vi "traitement cam A1.vi"(0 "ROI Carré 1":T1={"Global Rectangle"=[636, 369, 672, 405], "Contours"=[{"ID"=enum."External", "Type"=3, "Coordinates"=[636, 369, 672, 405]}]} {"Contours"."Type" items=["No Selection", "Point", "Line", "Rectangle", "Oval", "Polygon", "Freehand Region", "Annulus", "Unused2", "Unused3", "Broken Line", "Freehand Line", "Rotated Rectangle"]}, 7 "error in":errorcluster) -> (20 "Couleur carré 1":string[](array[string]), 27 "error out":errorcluster)   [LabVIEW 2019]
uses:
  <vilib>/vision/Classification.llb/IMAQ Classifier Read Options.ctl
  <vilib>/vision/NI_Vision_Development_Module.lvlib
panel:
  out "Couleur carré 12":string[](array[string])
  out "Couleur carré 11":string[](array[string])
  out "Couleur carré 10":string[](array[string])
  out "Couleur carré 9":string[](array[string])
  out "Couleur carré 8":string[](array[string])
  out "Couleur carré 7":string[](array[string])
  out "Couleur carré 6":string[](array[string])
  out "Couleur carré 5":string[](array[string])
  out "Couleur carré 4":string[](array[string])
  out "Couleur carré 3":string[](array[string])
  out "Couleur carré 2":string[](array[string])
  in  "ROI Carré 12":T1={"Global Rectangle"=[636, 369, 672, 405], "Contours"=[{"ID"=enum."External", "Type"=3, "Coordinates"=[636, 369, 672, 405]}]} {"Contours"."Type" items=["No Selection", "Point", "Line", "Rectangle", "Oval", "Polygon", "Freehand Region", "Annulus", "Unused2", "Unused3", "Broken Line", "Freehand Line", "Rotated Rectangle"]}
  in  "ROI Carré 11":T1={"Global Rectangle"=[636, 369, 672, 405], "Contours"=[{"ID"=enum."External", "Type"=3, "Coordinates"=[636, 369, 672, 405]}]} {"Contours"."Type" items=["No Selection", "Point", "Line", "Rectangle", "Oval", "Polygon", "Freehand Region", "Annulus", "Unused2", "Unused3", "Broken Line", "Freehand Line", "Rotated Rectangle"]}
  in  "ROI Carré 10":T1={"Global Rectangle"=[636, 369, 672, 405], "Contours"=[{"ID"=enum."External", "Type"=3, "Coordinates"=[636, 369, 672, 405]}]} {"Contours"."Type" items=["No Selection", "Point", "Line", "Rectangle", "Oval", "Polygon", "Freehand Region", "Annulus", "Unused2", "Unused3", "Broken Line", "Freehand Line", "Rotated Rectangle"]}
  in  "ROI Carré 9":T1={"Global Rectangle"=[636, 369, 672, 405], "Contours"=[{"ID"=enum."External", "Type"=3, "Coordinates"=[636, 369, 672, 405]}]} {"Contours"."Type" items=["No Selection", "Point", "Line", "Rectangle", "Oval", "Polygon", "Freehand Region", "Annulus", "Unused2", "Unused3", "Broken Line", "Freehand Line", "Rotated Rectangle"]}
  in  "ROI Carré 8":T1={"Global Rectangle"=[636, 369, 672, 405], "Contours"=[{"ID"=enum."External", "Type"=3, "Coordinates"=[636, 369, 672, 405]}]} {"Contours"."Type" items=["No Selection", "Point", "Line", "Rectangle", "Oval", "Polygon", "Freehand Region", "Annulus", "Unused2", "Unused3", "Broken Line", "Freehand Line", "Rotated Rectangle"]}
  in  "ROI Carré 7":T1={"Global Rectangle"=[636, 369, 672, 405], "Contours"=[{"ID"=enum."External", "Type"=3, "Coordinates"=[636, 369, 672, 405]}]} {"Contours"."Type" items=["No Selection", "Point", "Line", "Rectangle", "Oval", "Polygon", "Freehand Region", "Annulus", "Unused2", "Unused3", "Broken Line", "Freehand Line", "Rotated Rectangle"]}
  in  "ROI Carré 6":T1={"Global Rectangle"=[636, 369, 672, 405], "Contours"=[{"ID"=enum."External", "Type"=3, "Coordinates"=[636, 369, 672, 405]}]} {"Contours"."Type" items=["No Selection", "Point", "Line", "Rectangle", "Oval", "Polygon", "Freehand Region", "Annulus", "Unused2", "Unused3", "Broken Line", "Freehand Line", "Rotated Rectangle"]}
  in  "ROI Carré 5":T1={"Global Rectangle"=[636, 369, 672, 405], "Contours"=[{"ID"=enum."External", "Type"=3, "Coordinates"=[636, 369, 672, 405]}]} {"Contours"."Type" items=["No Selection", "Point", "Line", "Rectangle", "Oval", "Polygon", "Freehand Region", "Annulus", "Unused2", "Unused3", "Broken Line", "Freehand Line", "Rotated Rectangle"]}
  in  "ROI Carré 4":T1={"Global Rectangle"=[636, 369, 672, 405], "Contours"=[{"ID"=enum."External", "Type"=3, "Coordinates"=[636, 369, 672, 405]}]} {"Contours"."Type" items=["No Selection", "Point", "Line", "Rectangle", "Oval", "Polygon", "Freehand Region", "Annulus", "Unused2", "Unused3", "Broken Line", "Freehand Line", "Rotated Rectangle"]}
  in  "ROI Carré 3":T1={"Global Rectangle"=[636, 369, 672, 405], "Contours"=[{"ID"=enum."External", "Type"=3, "Coordinates"=[636, 369, 672, 405]}]} {"Contours"."Type" items=["No Selection", "Point", "Line", "Rectangle", "Oval", "Polygon", "Freehand Region", "Annulus", "Unused2", "Unused3", "Broken Line", "Freehand Line", "Rotated Rectangle"]}
  in  "ROI Carré 2":T1={"Global Rectangle"=[636, 369, 672, 405], "Contours"=[{"ID"=enum."External", "Type"=3, "Coordinates"=[636, 369, 672, 405]}]} {"Contours"."Type" items=["No Selection", "Point", "Line", "Rectangle", "Oval", "Polygon", "Freehand Region", "Annulus", "Unused2", "Unused3", "Broken Line", "Freehand Line", "Rotated Rectangle"]}
  out "Image Out":T2(plugin-control)
  # "C\nE\nN\nT\nR\nE\n\nR\nO\nU\nG\nE\nE"
  # "C\nE\nN\nT\nR\nE\n\nB\nL\nA\nN\nC"
  # "C\nE\nN\nT\nR\nE\n\nB\nL\nE\nU"
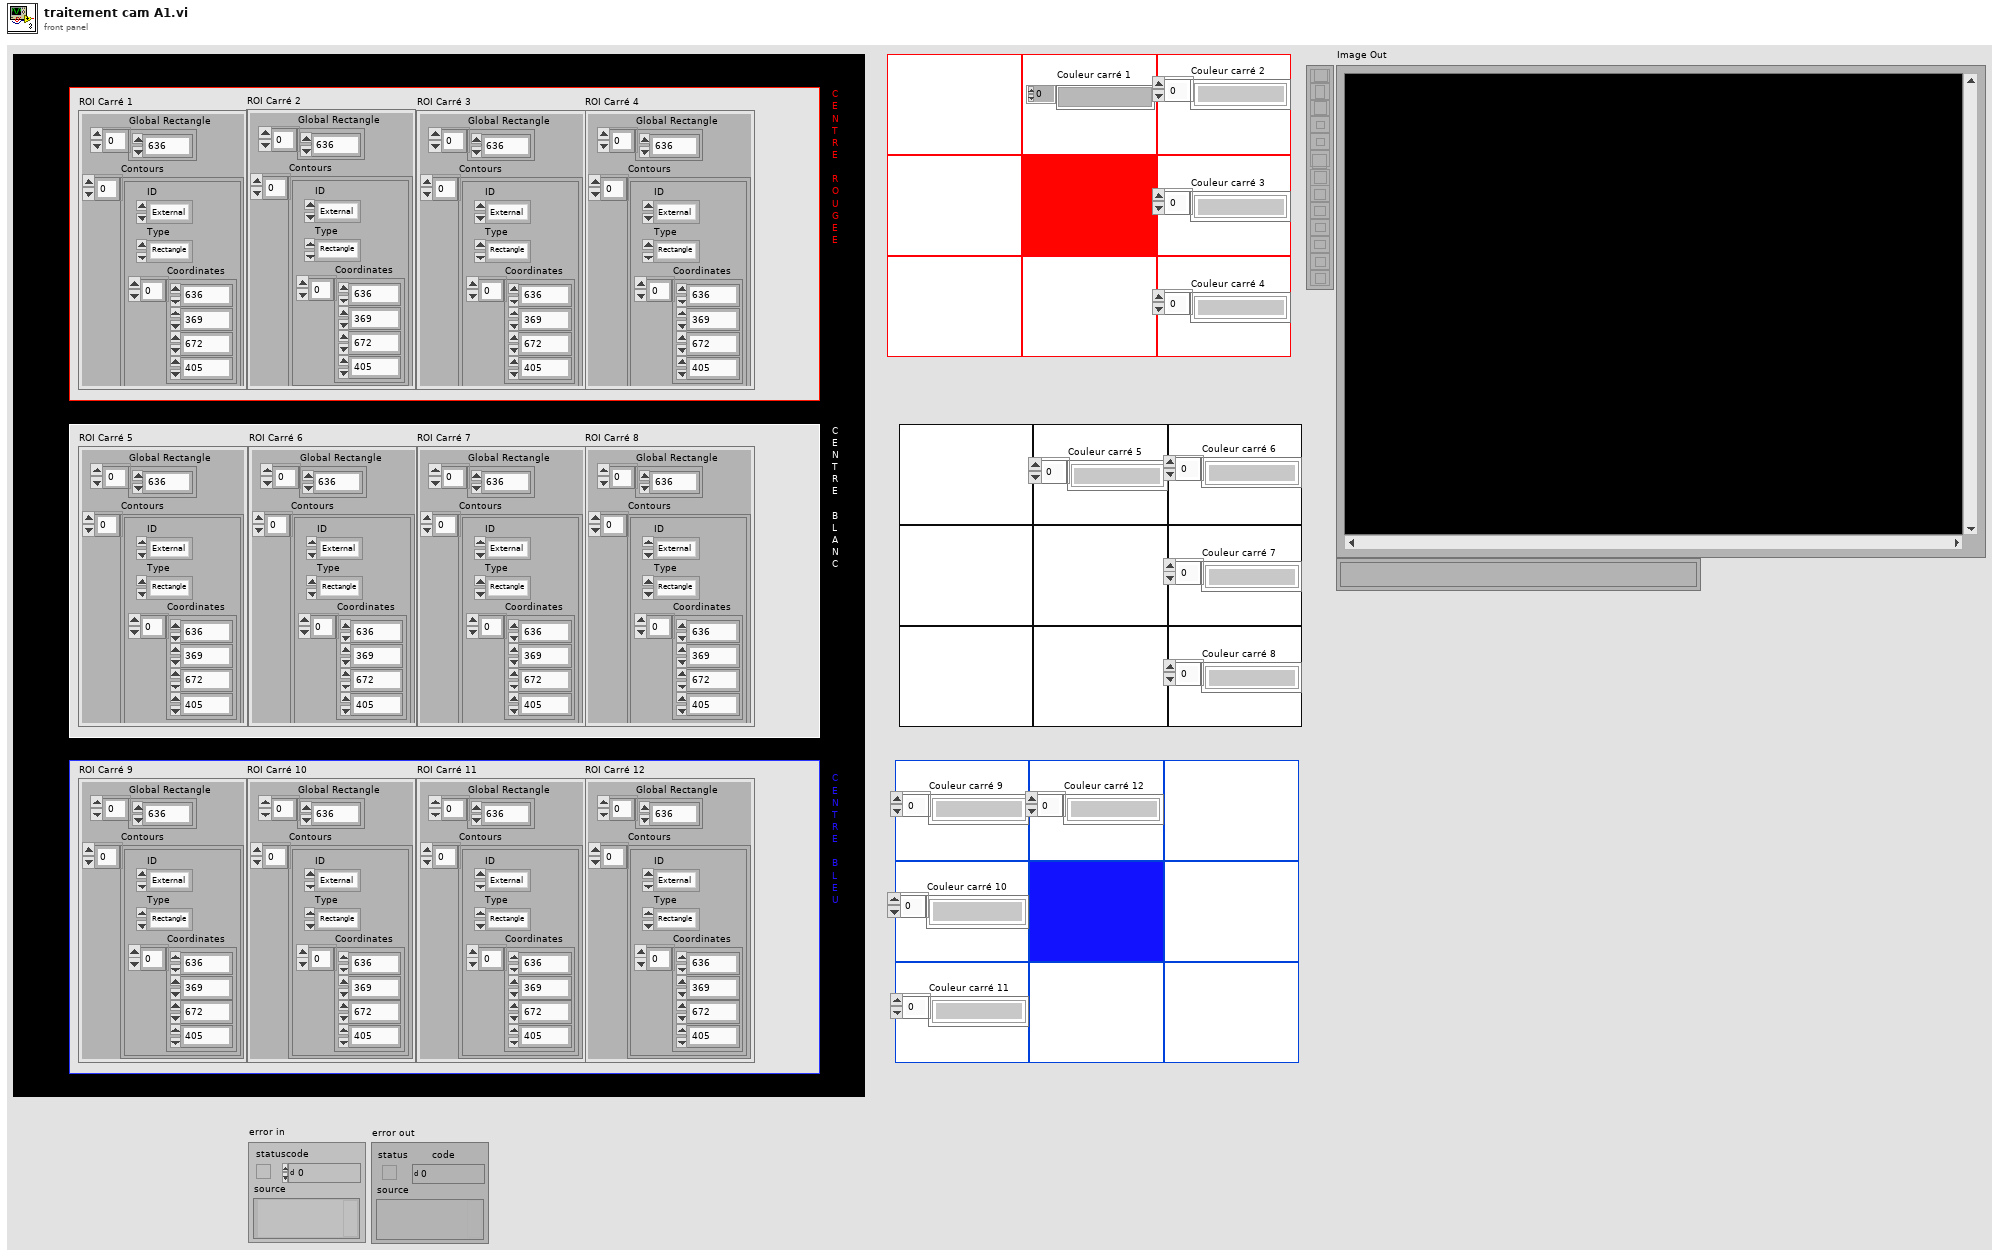
[diagram p1: front panel]
types:
  T1 = cluster{"Global Rectangle":i32[], "Contours":cluster{"ID":enum32{"External", "Internal"}, "Type":u32, "Coordinates":i32[]}[]}
  T2 = typedef "IMAQ Image.ctl" = refnum<image>
  T3 = typedef "IMAQ Classifier Read Options.ctl" = i32
  T4 = typedef "IMAQ Classifier Session.ctl" = refnum<k1>
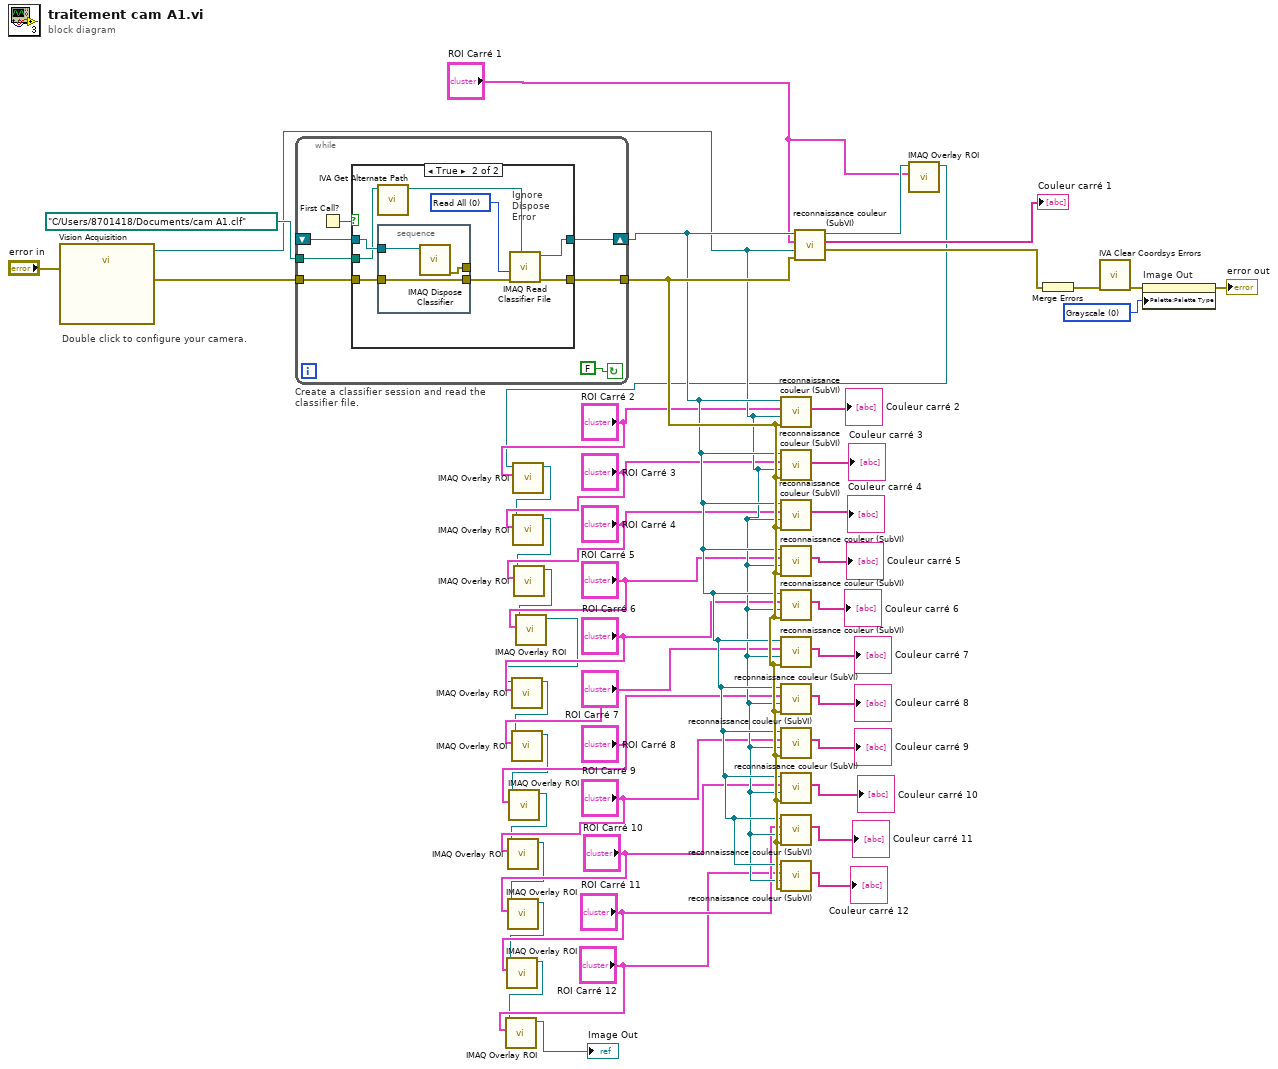
[diagram p0: block diagram]
diagram:
  w40 = u32 0 items=["Grayscale", "Binary", "Gradient", "Rainbow", "Temperature", "User Defined", "Binary 16 Bit", "Gradient 16 Bit", "Rainbow 16 Bit", "Temperature 16 Bit", "User Defined 16 Bit"] ("Palette Type")
  # "Double click to configure your camera."
  n1 = call "Vision Acquisition"("error in"="error in") -> ("Image Out"=w26:T2, "error out"=w45:errorcluster)  [unwired: 25 in]
  n2 = while "Create a classifier session and read the classifier file." {
    shift-right: [w55] -> w37
    shift-left: _ -> [w54]
    tunnel: w45 -> [w52]
    tunnel: [w51] -> w38
    tunnel: path "C:/Users/8701418/Documents/cam A1.clf" ("File Path") -> [w50]
    stop <- FALSE continue-if-true
    n3 = First Call?() -> (First Call?: T/F=w49:bool)
    n4 = case shown="True" w49 {
      tunnel: [w57 w64] -> w55
      tunnel: w54 -> [w57 w62]
      tunnel: w52 -> [w56 w61]
      tunnel: [w56 w63] -> w51
      tunnel: w50 -> [_ w59]
      frame False {
      }
      frame True {
        w65 = T3 0 items=["Read All", "Add Samples, Do Not Change Options", "Read Options, Do Not Add Samples"] ("Read Options")
        # "Ignore Dispose Error"
        n5 = call <vilib>:"IVA Get Alternate Path.vi"("Path In"=w59) -> ("Path Out"=w58:path)  [unwired: 10 out]
        n6 = stacked-sequence {
          tunnel: w62 -> [w68]
          tunnel: w61 -> [w67]
          tunnel: [w67] -> w60
          tunnel: [w66] -> _
          frame #0 {
            n7 = call "IMAQ Dispose Classifier"("Classifier Session"=w68) -> ("error out"=w66:errorcluster)  [unwired: 1 in, 9 out]
          }
        }
        n8 = call "IMAQ Read Classifier File"("File Path"=w58, "error in (no error)"=w60, "Read Options"=w65) -> ("error out"=w63:errorcluster, "Classifier Session"=w64:T4)  [unwired: 1 in, 6 out]
      }
    }
  }
  n9 = call "reconnaissance couleur (SubVI).vi"("error in (no error)"=w38, "Image Out in"=w26, "ROI Descriptor (Color Classification 1)"="ROI Carré 2", "Refnum in"=w37) -> ("Array 2"=→"Couleur carré 2":string[])  [unwired: 5 in, 2 out]
  n10 = call "reconnaissance couleur (SubVI).vi"("error in (no error)"=w38, "Image Out in"=w26, "ROI Descriptor (Color Classification 1)"="ROI Carré 3", "Refnum in"=w37) -> ("Array 2"=→"Couleur carré 3":string[])  [unwired: 5 in, 2 out]
  n11 = call "reconnaissance couleur (SubVI).vi"("error in (no error)"=w38, "Image Out in"=w26, "ROI Descriptor (Color Classification 1)"="ROI Carré 4", "Refnum in"=w37) -> ("Array 2"=→"Couleur carré 4":string[])  [unwired: 5 in, 2 out]
  n12 = call "reconnaissance couleur (SubVI).vi"("error in (no error)"=w38, "Image Out in"=w26, "ROI Descriptor (Color Classification 1)"="ROI Carré 5", "Refnum in"=w37) -> ("Array 2"=→"Couleur carré 5":string[])  [unwired: 5 in, 2 out]
  n13 = call "reconnaissance couleur (SubVI).vi"("error in (no error)"=w38, "Image Out in"=w26, "ROI Descriptor (Color Classification 1)"="ROI Carré 6", "Refnum in"=w37) -> ("Array 2"=→"Couleur carré 6":string[])  [unwired: 5 in, 2 out]
  n14 = call "reconnaissance couleur (SubVI).vi"("error in (no error)"=w38, "Image Out in"=w26, "ROI Descriptor (Color Classification 1)"="ROI Carré 7", "Refnum in"=w37) -> ("Array 2"=→"Couleur carré 7":string[])  [unwired: 5 in, 2 out]
  n15 = call "reconnaissance couleur (SubVI).vi"("error in (no error)"=w38, "Image Out in"=w26, "ROI Descriptor (Color Classification 1)"="ROI Carré 8", "Refnum in"=w37) -> ("Array 2"=→"Couleur carré 8":string[])  [unwired: 5 in, 2 out]
  n16 = call "reconnaissance couleur (SubVI).vi"("error in (no error)"=w38, "Image Out in"=w26, "ROI Descriptor (Color Classification 1)"="ROI Carré 9", "Refnum in"=w37) -> ("Array 2"=→"Couleur carré 9":string[])  [unwired: 5 in, 2 out]
  n17 = call "reconnaissance couleur (SubVI).vi"("error in (no error)"=w38, "Image Out in"=w26, "ROI Descriptor (Color Classification 1)"="ROI Carré 10", "Refnum in"=w37) -> ("Array 2"=→"Couleur carré 10":string[])  [unwired: 5 in, 2 out]
  n18 = call "reconnaissance couleur (SubVI).vi"("error in (no error)"=w38, "Image Out in"=w26, "ROI Descriptor (Color Classification 1)"="ROI Carré 11", "Refnum in"=w37) -> ("Array 2"=→"Couleur carré 11":string[])  [unwired: 5 in, 2 out]
  n19 = call "reconnaissance couleur (SubVI).vi"("error in (no error)"=w38, "Image Out in"=w26, "ROI Descriptor (Color Classification 1)"="ROI Carré 12", "Refnum in"=w37) -> ("Array 2"=→"Couleur carré 12":string[])  [unwired: 5 in, 2 out]
  n20 = call "reconnaissance couleur (SubVI).vi"("error in (no error)"=w38, "Image Out in"=w26, "ROI Descriptor (Color Classification 1)"="ROI Carré 1", "Refnum in"=w37) -> ("Array"=w44:errorcluster[], "Array 2"=→"Couleur carré 1":string[], "Refnum out"=w25:T2)  [unwired: 5 in]
  n21 = call "IMAQ Overlay ROI"("ROI Descriptor"="ROI Carré 1", "Image"=w25) -> ("Image Out"=w22:T2)  [unwired: 8 in, 1 out]
  n22 = call "IMAQ Overlay ROI"("ROI Descriptor"="ROI Carré 2", "Image"=w22) -> ("Image Out"=w11:T2)  [unwired: 8 in, 1 out]
  n23 = call "IMAQ Overlay ROI"("ROI Descriptor"="ROI Carré 3", "Image"=w11) -> ("Image Out"=w10:T2)  [unwired: 8 in, 1 out]
  n24 = call "IMAQ Overlay ROI"("ROI Descriptor"="ROI Carré 4", "Image"=w10) -> ("Image Out"=w9:T2)  [unwired: 8 in, 1 out]
  n25 = call "IMAQ Overlay ROI"("ROI Descriptor"="ROI Carré 5", "Image"=w9) -> ("Image Out"=w8:T2)  [unwired: 8 in, 1 out]
  n26 = call "IMAQ Overlay ROI"("ROI Descriptor"="ROI Carré 6", "Image"=w8) -> ("Image Out"=w7:T2)  [unwired: 8 in, 1 out]
  n27 = call "IMAQ Overlay ROI"("ROI Descriptor"="ROI Carré 7", "Image"=w7) -> ("Image Out"=w6:T2)  [unwired: 8 in, 1 out]
  n28 = call "IMAQ Overlay ROI"("ROI Descriptor"="ROI Carré 8", "Image"=w6) -> ("Image Out"=w5:T2)  [unwired: 8 in, 1 out]
  n29 = call "IMAQ Overlay ROI"("ROI Descriptor"="ROI Carré 9", "Image"=w5) -> ("Image Out"=w4:T2)  [unwired: 8 in, 1 out]
  n30 = call "IMAQ Overlay ROI"("ROI Descriptor"="ROI Carré 10", "Image"=w4) -> ("Image Out"=w3:T2)  [unwired: 8 in, 1 out]
  n31 = call "IMAQ Overlay ROI"("ROI Descriptor"="ROI Carré 11", "Image"=w3) -> ("Image Out"=w2:T2)  [unwired: 8 in, 1 out]
  n32 = call "IMAQ Overlay ROI"("ROI Descriptor"="ROI Carré 12", "Image"=w2) -> ("Image Out"=→"Image Out":T2)  [unwired: 8 in, 1 out]
  n33 = Merge Errors(w44) -> (w43:errorcluster)
  n34 = call <vilib>:"IVA Clear Coordsys Errors.vi"("error in (no error)"=w43) -> ("error out"=w42:errorcluster)  [unwired: 10 in]
  n35 = property on="Image Out" class="ImageControl"(error in=w42, "Palette:Palette Type"=w40) -> (error out=→"error out":errorcluster)  [unwired: 1 in, 1 out]
